vi "Write AttMap.vi"(8 "error in (no error)":errorcluster, 10 "AttMap":map{string, string}(c390), 11 "Node in":refnum<class "Node.lvclass">) -> (0 "error out":errorcluster, 3 "Node out":refnum<class "Node.lvclass">)   [LabVIEW 2025, in "Node.lvclass"]
uses:
  Node.lvclass
  Node.lvclass/Node.ctl
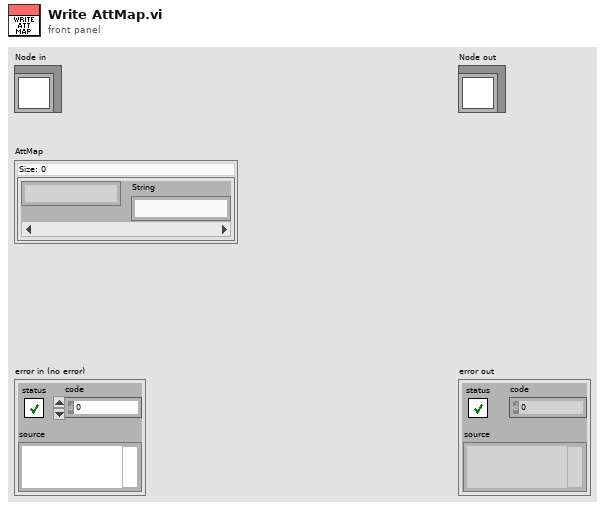
[diagram p1: front panel]
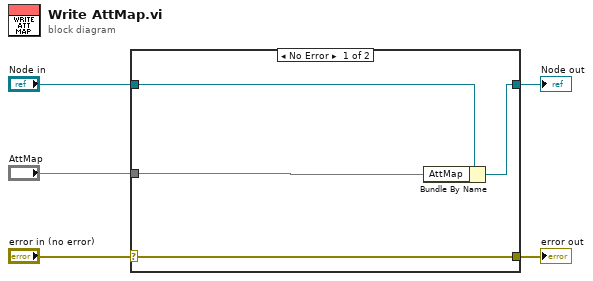
[diagram p0: block diagram]
diagram:
  n1 = case shown="No Error" "error in (no error)" {
    selector: "error in (no error)" -> [w9 w10]
    tunnel: [w9 w10] -> w4
    tunnel: [w7 w11] -> w2
    tunnel: "Node in" -> [w8 w11]
    tunnel: "AttMap" -> [w6 _]
    frame No Error {
      n2 = Bundle By Name(cluster=w8, "AttMap"=w6) -> (w7:refnum<class "Node.lvclass">)
    }
    frame Error {
    }
  }
  "error out" <- w4
  "Node out" <- w2
